vi "template.commit_id.vi"(8 "error in":errorcluster, 11 "Template in":refnum<class "Template.lvclass">) -> (0 "error out":errorcluster, 3 "Template out":refnum<class "Template.lvclass">)   [LabVIEW 2020, in "Template.lvclass"]
doc: "Returns the ID of this template's version (commit)."
uses:
  Template.lvclass
  Template.lvclass/Template.ctl
  client.lvlib
panel:
  out "out_needed out":u32
  out "commit id":string
  in  "buf":string
  in  "cap":u32
  in  "out_needed":u32
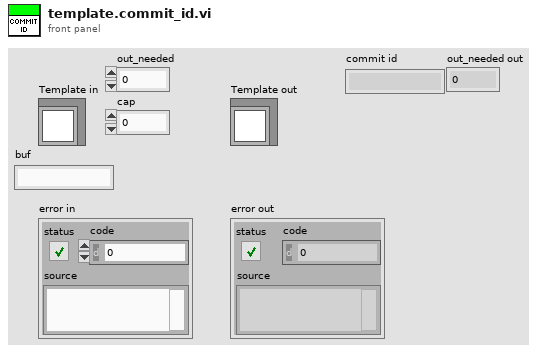
[diagram p1: front panel]
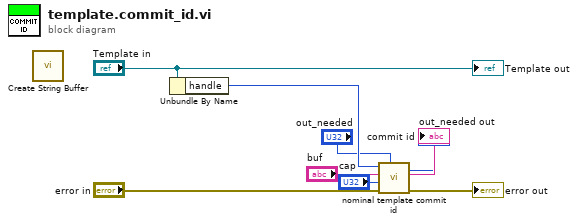
[diagram p0: block diagram]
diagram:
  n1 = call "Create String Buffer.vi"() -> ()  [unwired: 9 in, 3 out]
  n2 = Unbundle By Name("Template in") -> ("handle"=w7:i32)
  n3 = call "nominal template commit id.vi"("out_needed"="out_needed", "error in (no error)"="error in", "cap"="cap", "buf"="buf", "template_"=w7) -> ("error out"=→"error out":errorcluster, "buf out"=→"commit id":string, "out_needed out"=→"out_needed out":u32)  [unwired: 3 in, 1 out]
  "Template out" <- "Template in"
